vi "ConnectedStatus.vi"(8 "error in (no error)":errorcluster, 11 "ChromaPowerSupplyModel in":refnum<class "ChromaPowerSupplyModel.lvclass">) -> (0 "error out":errorcluster, 2 "Any Connections":bool, 3 "ChromaPowerSupplyModel out":refnum<class "ChromaPowerSupplyModel.lvclass">)   [LabVIEW 2018, in "AcPwrPlugins.lvlib" / "ChromaPowerSupplyModel.lvclass"]
doc: "This VI checks if the instrument has been connected and reports that value to any function calling it."
uses:
  ChromaPowerSupplyModel.lvclass
  AcPwrBaseClass/AcPwrBase.lvclass
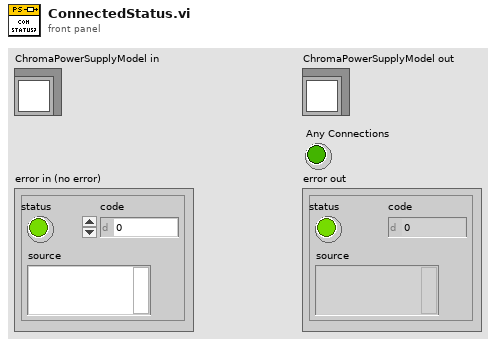
[diagram p1: front panel]
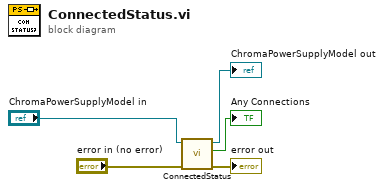
[diagram p0: block diagram]
diagram:
  n1 = call-parent "ConnectedStatus.vi"("error in (no error)"="error in (no error)", "AcPwrBase in"="ChromaPowerSupplyModel in") -> ("error out"=→"error out":errorcluster, "Any Connections"=→"Any Connections":bool, "AcPwrBase out"=→"ChromaPowerSupplyModel out":refnum<class "ChromaPowerSupplyModel.lvclass">)  [unwired: 7 in]
